vi "Launch Module.vi"(8 "error in (no error)":errorcluster, 9 "params":variant, 11 "Controller in":refnum<class "Controller.lvclass">) -> (0 "error out":errorcluster, 3 "Controller out":refnum<class "Controller.lvclass">)   [LabVIEW 2020, in "Controller.lvclass"]
uses:
  Controller.lvclass
  controls/Module Launch Data.ctl
  Module/Module.lvclass
  controls/Request.ctl
  Controller.lvclass/Controller.ctl
  Module/Module.lvclass/Module.ctl
  Module/Properties/Read Name.vi
  Properties/Read E-Stop.vi
  Properties/Read Globals.vi
  Properties/Read ResponseAvailable.vi
  Module/Properties/Write E-Stop.vi
  Module/Properties/Write Globals.vi
  Module/Properties/Write Response.vi
  Module/Properties/Write Name.vi
  Module/Properties/Write MQ.vi
  <vilib>/ErrorRing/Error Ring.xnode
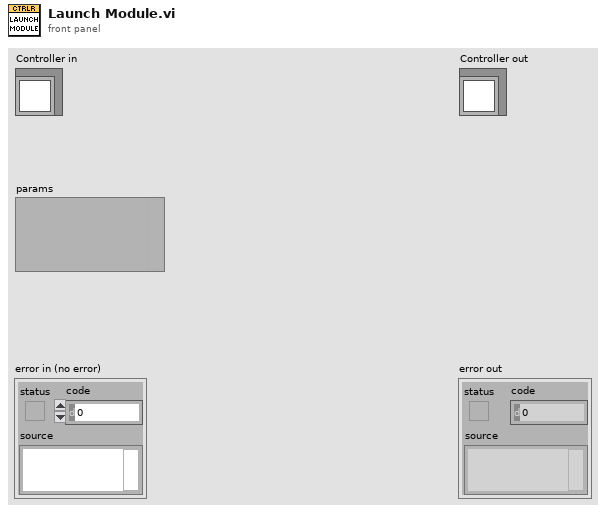
[diagram p1: front panel]
types:
  T1 = typedef "Module Launch Data.ctl" = cluster{"Path":string, "Name":string, "FrontPanel":bool}
  T2 = enum32{"Invalid", "Standard", "Closed", "Hidden", "Minimized", "Maximized"}
  T3 = typedef "Request.ctl" = cluster{"Method":string, "Params":variant}
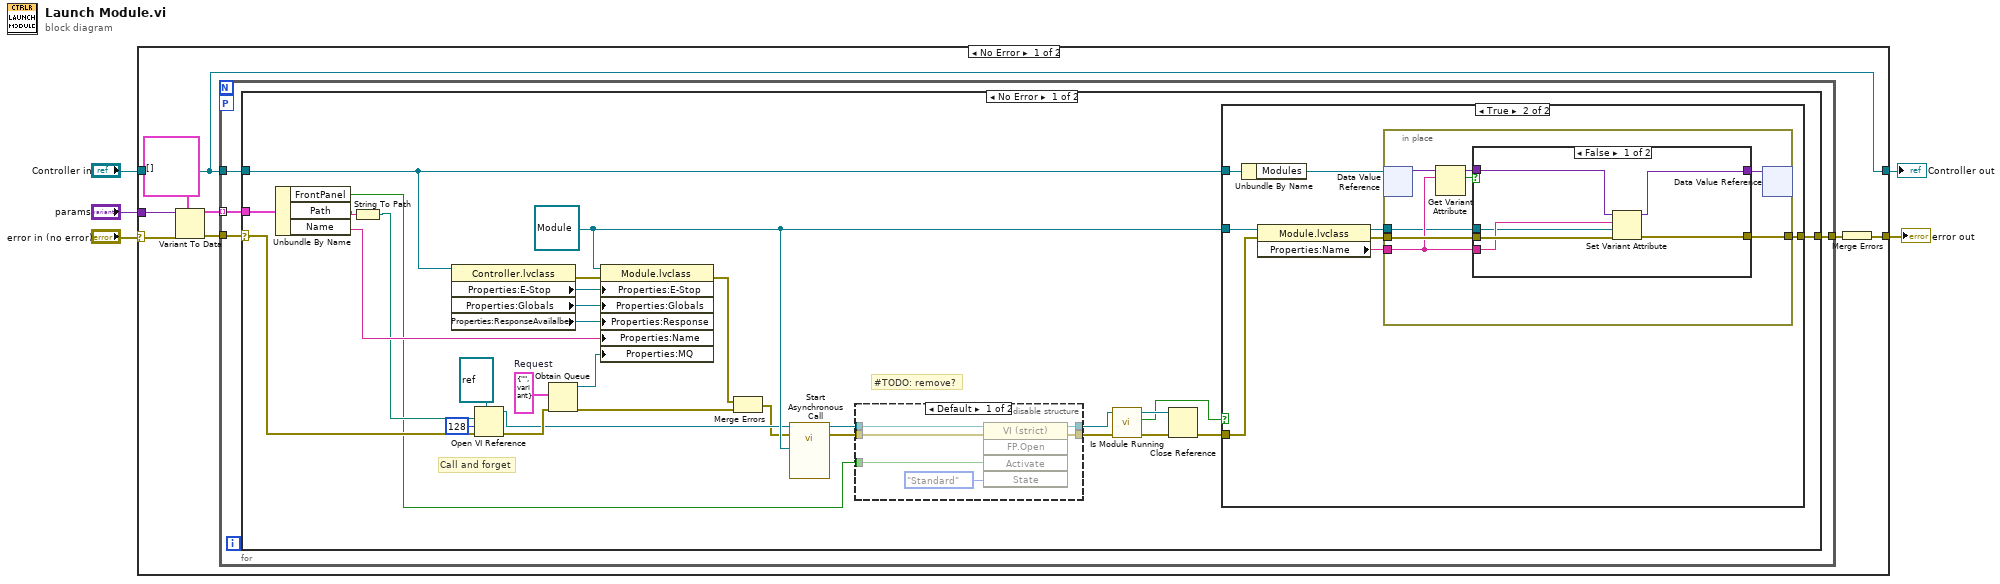
[diagram p0: block diagram]
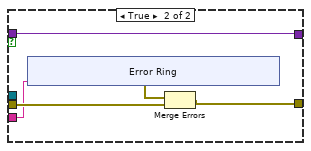
[diagram p4: hidden frame]
diagram:
  n1 = case shown="No Error" "error in (no error)" {
    selector: "error in (no error)" -> [w11 w91]
    tunnel: [w6 w91] -> w4
    tunnel: [w13 w90] -> w2
    tunnel: "Controller in" -> [w13 w90]
    tunnel: "params" -> [w9 _]
    frame No Error {
      n2 = Variant To Data(error in=w11, type=T1[] [] ("Module Info"), Variant=w9) -> (data=w8:T1[], error out=w10:errorcluster)
      n3 = for {
        tunnel: w13 -> [w17]
        tunnel: w8 -> [w16] mode=indexing
        tunnel: w10 -> [w14]
        tunnel: [w15] -> _ mode=indexing
        workers-P: _ -> [_]
        tunnel: [w15] -> w7
        n4 = case shown="No Error" w14 {
          selector: w14 -> [w20 w89]
          tunnel: w17 -> [w47 _]
          tunnel: w16 -> [w43 _]
          tunnel: [w42 w89] -> w15
          frame No Error {
            w40 = refnum<class "Module.lvclass"> refnum ("Module in")
            w36 = T3 {"Method"="", "Params"=variant}  # Request
            # "#TODO: remove?"
            # "Call and forget"
            n5 = Unbundle By Name(w43) -> ("FrontPanel"=w18:bool, "Path"=w45:string, "Name"=w46:string)
            n6 = String To Path(string=w45) -> (path=w44:path)
            n7 = property class="Controller.lvclass"(reference=w47) -> (error out=w28:errorcluster, "Properties:E-Stop"=w24:refnum<user-event>, "Properties:Globals"=w23:refnum<data-value>, "Properties:ResponseAvailalbe"=w22:refnum<user-event>)  [unwired: 1 in, 1 out]
            n8 = Open VI Reference(type specifier VI Refnum (for type only)=refnum<vi> refnum, vi path=w44, options=128, error in (no error)=w20) -> (vi reference=w35:refnum<vi>, error out=w37:errorcluster)  [unwired: 2 in]
            n9 = Obtain Queue(element data type=w36, error in (no error)=w37) -> (queue out=w21:refnum<queue>, error out=w26:errorcluster)  [unwired: 3 in, 1 out]
            n10 = property class="Module.lvclass"(reference=w40, error in=w28, "Properties:E-Stop"=w24, "Properties:Globals"=w23, "Properties:Response"=w22, "Properties:Name"=w46, "Properties:MQ"=w21) -> (error out=w25:errorcluster)  [unwired: 1 out]
            n11 = Merge Errors(w25, w26) -> (w27:errorcluster)
            n12 = call-by-ref "Start Asynchronous Call"(reference=w35, error in=w27, "Module in"=w40) -> (reference out=w32:refnum<vi>, error out=w33:errorcluster)  [unwired: 11 in]
            n13 = disable-structure shown="Default" {
              disable-tunnel: w33 -> [w53 w55]
              disable-tunnel: w32 -> [w52 w54]
              disable-tunnel: [w50 w55] -> w38
              disable-tunnel: [w49 w54] -> w31
              disable-tunnel: w18 -> [w48 _]
              frame condition #0 {
                n14 = invoke class="VI (strict)" method="FP.Open"(reference=w52, error in=w53, "Activate"=w48, "State"=T2."Standard") -> (reference out=w49:refnum<vi>, error out=w50:errorcluster)  [unwired: 1 in, 3 out]
              }
              frame condition #1 (active) {
              }
            }
            n15 = call "Is Module Running.vi"("error in (no error)"=w38, "VI reference in"=w31) -> ("error out"=w30:errorcluster, "Is Running?"=w19:bool, "VI reference out"=w29:refnum<vi>)  [unwired: 6 in, 1 out]
            n16 = Close Reference(reference=w29, error in (no error)=w30) -> (error out=w41:errorcluster)
            n17 = case shown="True" w19 {
              tunnel: w47 -> [_ w64]
              tunnel: w41 -> [w56 w63]
              tunnel: [w56 w62] -> w42
              tunnel: w40 -> [_ w57]
              frame False {
              }
              frame True {
                n18 = Unbundle By Name(w64) -> ("Modules"=w61:refnum<data-value>)
                n19 = property class="Module.lvclass"(reference=w57, error in=w63) -> (reference out=w58:refnum<class "Module.lvclass">, error out=w59:errorcluster, "Properties:Name"=w60:string)
                n20 = in-place {
                  in-place-border: w60 -> [w68]
                  in-place-border: w59 -> [w71]
                  in-place-border: w58 -> [w67]
                  in-place-border: [w70] -> w62
                  n21 = in-place-dvr #1(w61) -> (w69:variant)  [unwired: 1 out]
                  n22 = Get Variant Attribute(Variant=w69, name=w68) -> (duplicate Variant=w66:variant, found=w65:bool)  [unwired: 2 in, 2 out]
                  n23 = case shown="False" w65 {
                    tunnel: [w78 w83] -> w72
                    tunnel: w71 -> [w77 w81]
                    tunnel: [w76 w82] -> w70
                    tunnel: w68 -> [w75 w80]
                    tunnel: w67 -> [w74 _]
                    tunnel: w66 -> [w73 w83]
                    frame False {
                      n24 = Set Variant Attribute(Variant=w73, name=w75, value=w74, error in=w77) -> (Variant out=w78:variant, error out=w76:errorcluster)  [unwired: 1 out]
                    }
                    frame True {
                      n25 = xnode "Error Ring"("parameter 0"=w80) -> ("error out"=w79:errorcluster)
                      n26 = Merge Errors(w79, w81) -> (w82:errorcluster)
                    }
                  }
                  n27 = in-place-dvr #1(w72) -> ()  [unwired: 2 out]
                }
              }
            }
          }
          frame Error {
          }
        }
      }
      n28 = Merge Errors(w7) -> (w6:errorcluster)
    }
    frame Error {
    }
  }
  "error out" <- w4
  "Controller out" <- w2
